vi "Working with Variants.vi"() -> ()   [LabVIEW 2015]
uses:
  <vilib>/NI/JSON Support for LabVIEW/JSON Data Classes/JSON Datatype/JSON Null.lvclass
  <vilib>/NI/JSON Support for LabVIEW/JSON Data Classes/JSON Helper/JSON Helper.lvclass
panel:
  out "data 5":T1
  in  "Cluster":T1
  out "JSON Object":string
  out "JSON Numeric Array":string
  out "data 4":dbl[](array[numeric])
  in  "Numeric Array":dbl[](array[numeric]) format="%#_13g"
  out "data 3":bool
  in  "Boolean":bool=TRUE
  out "JSON Booelan":string
  in  "Numeric":dbl=12.0 format="%#_13g"
  in  "String":string="Hello World"
  out "data 2":dbl
  out "JSON Numeric":string
  out "data":string
  out "JSON String":string
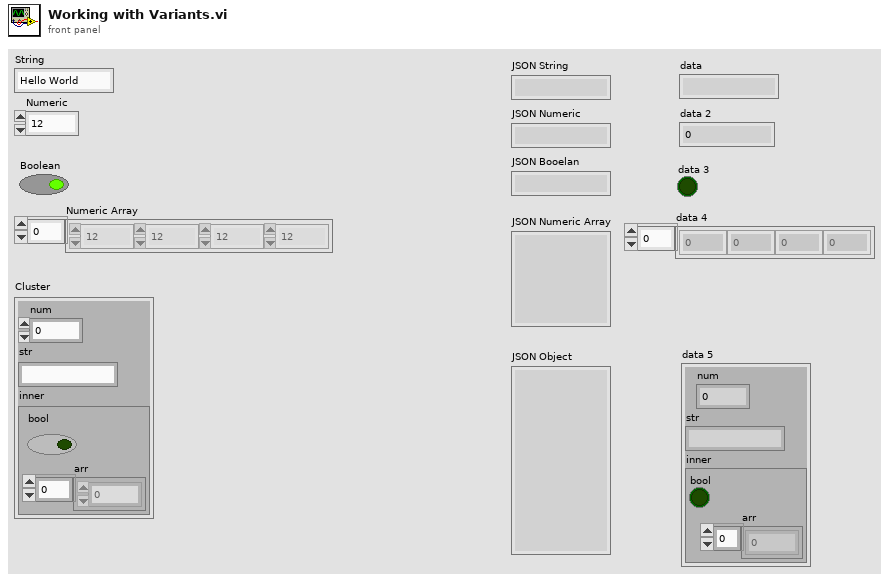
[diagram p1: front panel]
types:
  T1 = cluster{"num":dbl, "str":string, "inner":cluster{"bool":bool, "arr":dbl[]}}
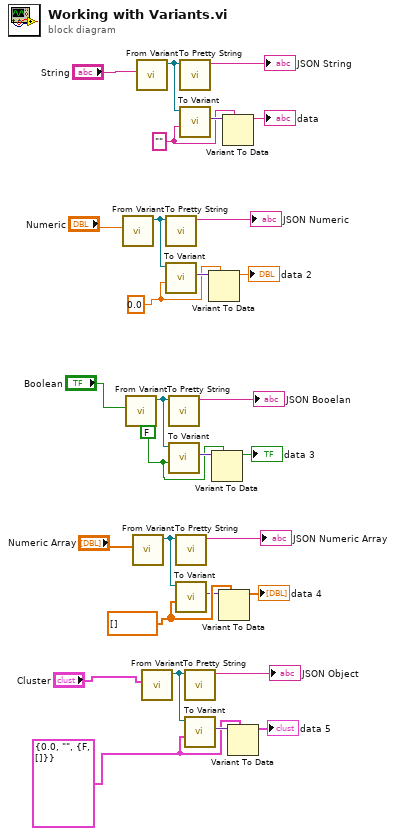
[diagram p0: block diagram]
diagram:
  w2 = T1 {"num"=0.0, "str"="", "inner"={"bool"=FALSE, "arr"=[]}} ("outer")
  w11 = dbl[] []
  w14 = FALSE ("Boolean")
  w20 = 0.0
  w26 = ""
  n1 = call <vilib>:"From Variant.vi"("Variant"="Numeric") -> ("JSON out"=w22:refnum<class "JSON Null.lvclass">)  [unwired: 9 in, 1 out]
  n2 = call <vilib>:"From Variant.vi"("Variant"="Boolean") -> ("JSON out"=w18:refnum<class "JSON Null.lvclass">)  [unwired: 9 in, 1 out]
  n3 = call <vilib>:"From Variant.vi"("Variant"="Numeric Array") -> ("JSON out"=w9:refnum<class "JSON Null.lvclass">)  [unwired: 9 in, 1 out]
  n4 = call <vilib>:"From Variant.vi"("Variant"="String") -> ("JSON out"=w30:refnum<class "JSON Null.lvclass">)  [unwired: 9 in, 1 out]
  n5 = call <vilib>:"From Variant.vi"("Variant"="Cluster") -> ("JSON out"=w4:refnum<class "JSON Null.lvclass">)  [unwired: 9 in, 1 out]
  n6 = call-dynamic "To Pretty String.vi"("JSON Datatype in"=w22) -> ("Pretty Print String"=→"JSON Numeric":string)  [unwired: 9 in, 1 out]
  n7 = call <vilib>:"To Variant.vi"("datatype and defaults"=w20, "JSON Datatype in"=w22) -> ("Variant"=w24:variant)  [unwired: 7 in, 2 out]
  n8 = call-dynamic "To Pretty String.vi"("JSON Datatype in"=w18) -> ("Pretty Print String"=→"JSON Booelan":string)  [unwired: 9 in, 1 out]
  n9 = call <vilib>:"To Variant.vi"("datatype and defaults"=w14, "JSON Datatype in"=w18) -> ("Variant"=w16:variant)  [unwired: 7 in, 2 out]
  n10 = call-dynamic "To Pretty String.vi"("JSON Datatype in"=w9) -> ("Pretty Print String"=→"JSON Numeric Array":string)  [unwired: 9 in, 1 out]
  n11 = call <vilib>:"To Variant.vi"("datatype and defaults"=w11, "JSON Datatype in"=w9) -> ("Variant"=w7:variant)  [unwired: 7 in, 2 out]
  n12 = call-dynamic "To Pretty String.vi"("JSON Datatype in"=w30) -> ("Pretty Print String"=→"JSON String":string)  [unwired: 9 in, 1 out]
  n13 = call <vilib>:"To Variant.vi"("datatype and defaults"=w26, "JSON Datatype in"=w30) -> ("Variant"=w27:variant)  [unwired: 7 in, 2 out]
  n14 = call-dynamic "To Pretty String.vi"("JSON Datatype in"=w4) -> ("Pretty Print String"=→"JSON Object":string)  [unwired: 9 in, 1 out]
  n15 = call <vilib>:"To Variant.vi"("datatype and defaults"=w2, "JSON Datatype in"=w4) -> ("Variant"=w6:variant)  [unwired: 7 in, 2 out]
  n16 = Variant To Data(type=w20, Variant=w24) -> (data=→"data 2":dbl)  [unwired: 1 in, 1 out]
  n17 = Variant To Data(type=w14, Variant=w16) -> (data=→"data 3":bool)  [unwired: 1 in, 1 out]
  n18 = Variant To Data(type=w11, Variant=w7) -> (data=→"data 4":dbl[])  [unwired: 1 in, 1 out]
  n19 = Variant To Data(type=w26, Variant=w27) -> (data=→"data":string)  [unwired: 1 in, 1 out]
  n20 = Variant To Data(type=w2, Variant=w6) -> (data=→"data 5":T1)  [unwired: 1 in, 1 out]
